vi "DetectAnalyser.vi"(8 "error in (no error)":errorcluster, 11 "DemoMicrosope in":refnum<class "DemoMicrosope.lvclass">) -> (0 "error out":errorcluster, 3 "DemoMicrosope out":refnum<class "DemoMicrosope.lvclass">)   [LabVIEW 2020, in "DemoMicrosope.lvlib" / "DemoMicrosope.lvclass"]
uses:
  DemoMicrosope.lvclass
  Logic Layer/DataLogger/DataLogger/DataLogger.lvclass
  E:/Development/DevHardSoftware/MicroscopyFramework/Analyser/Analyser/Analyser.lvclass
  Hardware Abstraction Layer/Microscope/Microscope/Microscope.lvclass
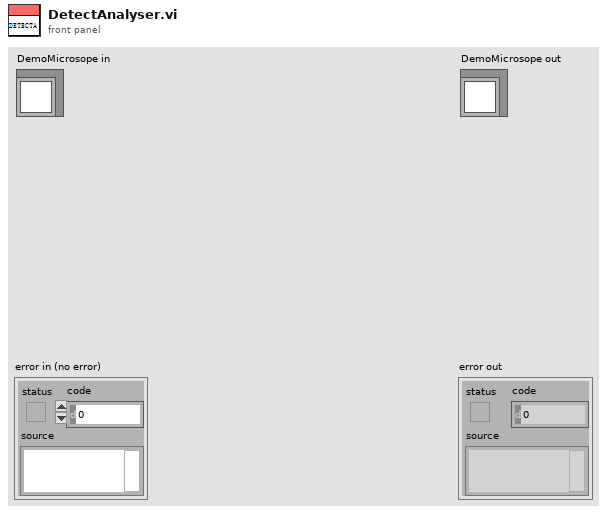
[diagram p1: front panel]
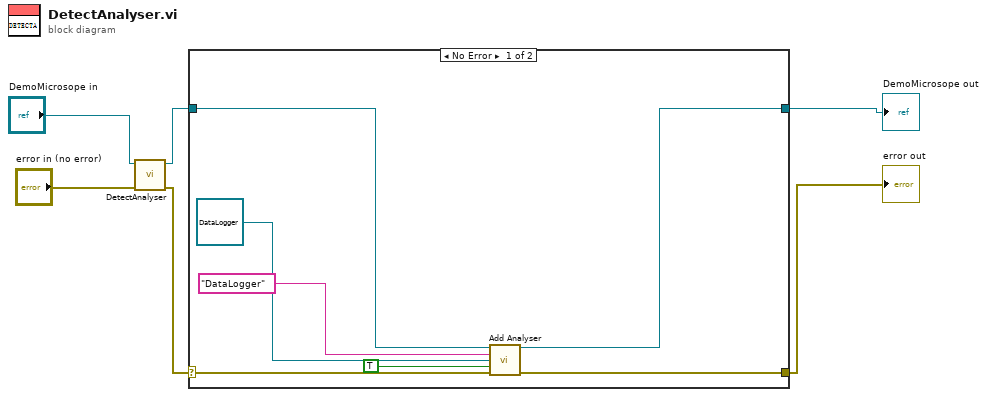
[diagram p0: block diagram]
diagram:
  n1 = call-parent "DetectAnalyser.vi"("error in (no error)"="error in (no error)", "Microscope in"="DemoMicrosope in") -> ("error out"=w3:errorcluster, "Microscope out"=w4:refnum<class "DemoMicrosope.lvclass">)  [unwired: 8 in]
  n2 = case shown="No Error" w3 {
    selector: w3 -> [w13 w15]
    tunnel: [w12 w15] -> w2
    tunnel: [w10 w14] -> w1
    tunnel: w4 -> [w11 w14]
    frame No Error {
      n3 = call-dynamic "Add Analyser.vi"("Microscope in"=w11, "Label"="DataLogger", "Analyser"=refnum<class "DataLogger.lvclass"> refnum ("DataLogger.lvlib:DataLogger.lvclass"), "RegisterInPipleline?(F)"=TRUE, "error in (no error)"=w13) -> ("Microscope out"=w10:refnum<class "DemoMicrosope.lvclass">, "error out"=w12:errorcluster)  [unwired: 7 in, 2 out]
    }
    frame Error {
    }
  }
  "error out" <- w2
  "DemoMicrosope out" <- w1
